vi "Pix2Pos.vi"(0 "Chemin vers le fichier PNG":path, 5 "entrée d'erreur":errorcluster) -> (14 "X1":dbl, 15 "Y1":dbl, 16 "X2":dbl, 17 "Y2":dbl, 18 "new picture":picture caption="nouvelle image", 19 "sortie d'erreur":errorcluster)   [LabVIEW 2017]
panel:
  out "Couleur 1":dbl
  out "Couleur 2":dbl
  out "Pos":string
  out "hauteur":i16
  out "largeur":i16
  out "image":u32[](array[numeric])
  out "image depth":i32
  out "standard output":string caption="sortie standard"
  out "Pixmap.bin":u32[](array[numeric])
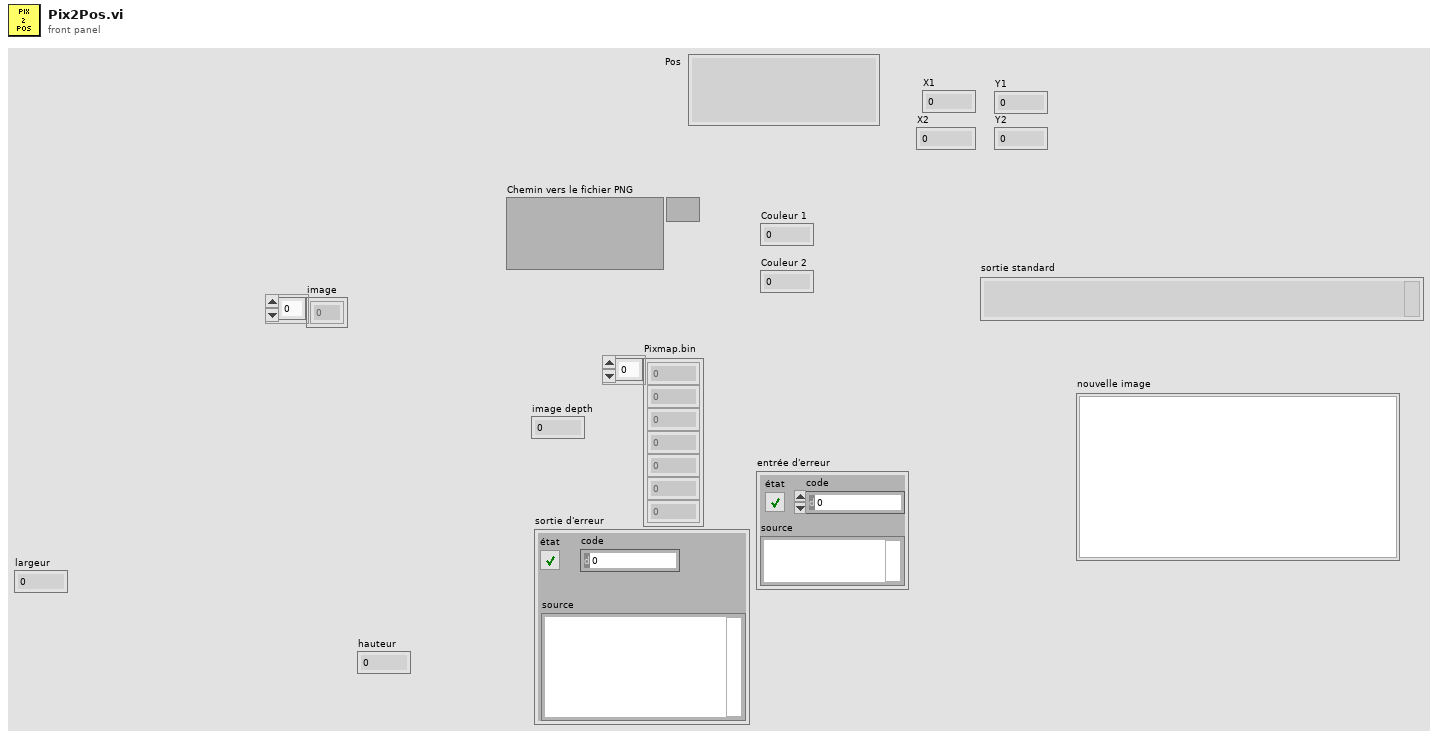
[diagram p1: front panel]
types:
  T1 = enum16{"big-endian, network order", "native, host order", "little-endian"}
  T2 = typedef "imagedata.ctl" = cluster{"image type":i32, "image depth":i32, "image":u8[], "mask":u8[], "colors":u32[], "Rectangle":cluster{"left":i16, "top":i16, "right":i16, "bottom":i16}}
  T3 = cluster{"[0]":dbl, "[1]":dbl, "[2]":dbl, "[3]":dbl, "[4]":dbl, "[5]":dbl, "[6]":dbl, "[7]":dbl, "[8]":dbl}
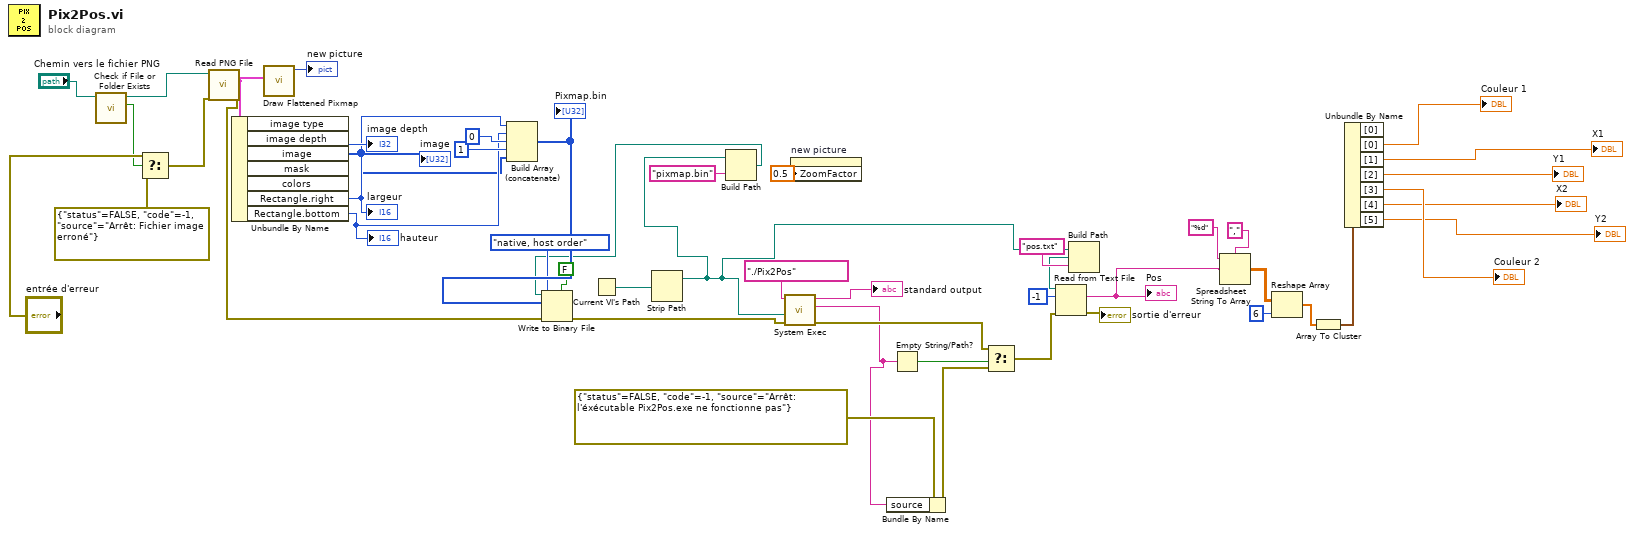
[diagram p0: block diagram]
diagram:
  n1 = call <vilib>:"Check if File or Folder Exists.vi"("path"="Chemin vers le fichier PNG") -> ("file or folder exists?"=w4:bool, "dup path"=w6:path)  [unwired: 8 in, 1 out]
  n2 = Select(t="entrée d'erreur", s=w4, f=errorcluster {"status"=FALSE, "code"=-1, "source"="Arrêt: Fichier image erroné"} ("constante d'erreur")) -> (s? t:f=w3:errorcluster)
  n3 = call <vilib>:"Read PNG File.vi"("error in (no error)"=w3, "path to PNG file"=w6) -> ("error out"=w2:errorcluster, "image data"=w38:T2)  [unwired: 7 in, 1 out]
  n4 = Unbundle By Name(w38) -> ("image depth"=→"image depth":i32, "image"=w33:u8[], "Rectangle.right"=w35:i16, "Rectangle.bottom"=w34:i16)  [unwired: 3 out]
  "image" <- w33
  "largeur" <- w35
  "hauteur" <- w34
  n5 = call <vilib>:"Draw Flattened Pixmap.vi"("image data"=w38) -> ("new picture"=→"new picture":picture)  [unwired: 8 in]
  n6 = Build Array (concatenate)(w35, w34, u32 0 ("color 1"), u32 1 ("color 2"), w33) -> (w47:u32[])
  "Pixmap.bin" <- w47
  n7 = Current VI's Path() -> (path=w43:path)
  n8 = Strip Path(path=w43) -> (stripped path=w27:path)  [unwired: 1 out]
  n9 = Build Path(base path=w27, name or relative path="pixmap.bin" ("nom ou chemin relatif")) -> (appended path=w29:path)
  n10 = Write to Binary File ("Écrire dans un fichier binaire")(file (use dialog)=w29, data=w47, error in=w2, 5:FALSE, 9:T1."native, host order" ("ordre des octets (0 : big-Endian, network order)")) -> (error out=w40:errorcluster)  [unwired: 1 in, 2 out]
  n11 = call <vilib>:"System Exec.vi"("error in (no error)"=w40, "working directory"=w27, "command line"="./Pix2Pos") -> ("error out"=w12:errorcluster, "standard error"=w9:string, "standard output"=→"standard output":string)  [unwired: 5 in, 1 out]
  n12 = property on="new picture" class="Pict"("ZoomFactor"=sgl 0.5 ("Facteur de zoom")) -> ()  [unwired: 2 in, 2 out]
  n13 = Bundle By Name(cluster=errorcluster {"status"=FALSE, "code"=-1, "source"="Arrêt: l'éxécutable Pix2Pos.exe ne fonctionne pas"} ("f"), "source"=w9) -> (w8:errorcluster)
  n14 = Empty String/Path?(string/path=w9) -> (empty?=w13:bool)
  n15 = Select(t=w12, s=w13, f=w8) -> (s? t:f=w11:errorcluster)
  n16 = Build Path(base path=w27, name or relative path="pos.txt" ("nom ou chemin relatif")) -> (appended path=w30:path)
  n17 = Read from Text File(file (use dialog)=w30, count=-1 ("nombre"), error in=w11) -> (text=w26:string, error out=→"sortie d'erreur":errorcluster)  [unwired: 1 in, 2 out]
  "Pos" <- w26
  n18 = Spreadsheet String To Array(delimiter (Tab)="," ("chaîne de format"), format string="%d" ("séparateur (Tabulation)"), spreadsheet string=w26) -> (array=w22:dbl[][])  [unwired: 1 in]
  n19 = Reshape Array(w22, 6 ("taille de la dimension")) -> (w23:dbl[])
  n20 = Array To Cluster(array=w23) -> (cluster=w20:T3)
  n21 = Unbundle By Name(w20) -> ("[0]"=→"Couleur 1":dbl, "[1]"=→"X1":dbl, "[2]"=→"Y1":dbl, "[3]"=→"Couleur 2":dbl, "[4]"=→"X2":dbl, "[5]"=→"Y2":dbl)  [unwired: 1 out]
